vi "darksider.vi"(8 "sum threshold":dbl, 9 "background":u16=1000, 10 "Frame Index start":i32=-1, 11 "Path":path) -> (0 "Edge 2":i32, 1 "Edge 1":i32, 2 "lateral position indexs":dbl[](array[numeric]), 3 "centroid":sgl[][](array[numeric]), 4 "Total Frames":i32, 6 "index of element":i32)   [LabVIEW 2021]
uses:
  <vilib>/Analysis/baseanly.llb/Mean (DBL).vi
  <vilib>/vision/NI_Vision_Development_Module.lvlib
  <vilib>/Analysis/NI_AALBase.lvlib
panel:
  out "lateral position indexsy":dbl[](array[numeric])
  out "size(s)":i32
  out "Waveform Graph 2":sgl[](graph)
  out "Particle Reports (Pixels)":T1(array[cluster]) {"Orientation" format="%.2f"; "Dimensions"."Height" format="%.2f"; "Dimensions"."Width" format="%.2f"; "Center of Mass"."Y" format="%.2f"; "Center of Mass"."X" format="%.2f"; "Bounding Rect"."Bottom" format="%.2f"; "Bounding Rect"."Right" format="%.2f"; "Bounding Rect"."Top" format="%.2f"; "Bounding Rect"."Left" format="%.2f"; "Number of Holes" format="%.2f"; "Area" format="%.2f"}
  in  "Selection Values 2":T3(array[cluster])=[{"Measurement Parameter"=1, "Range Lower Value"=200.0, "Range Upper Value"=1848.0, "Range"=FALSE, "Measurement Type"=FALSE}] {"Measurement Parameter" items=["Center of Mass X", "Center of Mass Y", "First Pixel X", "First Pixel Y", "Bounding Rect Left", "Bounding Rect Top", "Bounding Rect Right", "Bounding Rect Bottom", "Max Feret Diameter Start X", "Max Feret Diameter Start Y", "Max Feret Diameter End X", "Max Feret Diameter End Y", "Max Horiz. Segment Length Left", "Max Horiz. Segment Length Right", "Max Horiz. Segment Length Row", "-", "Bounding Rect Width", "Bounding Rect Height", "Bounding Rect Diagonal", "Perimeter", "Convex Hull Perimeter", "Holes' Perimeter", "Max Feret Diameter", "Equivalent Ellipse Major Axis", "Equivalent Ellipse Minor Axis", "Equivalent Ellipse Minor Axis (Feret)", "Equivalent Rect Long Side", "Equivalent Rect Short Side", "Equivalent Rect Diagonal", "Equivalent Rect Short Side (Feret)", "Average Horiz. Segment Length", "Average Vert. Segment Length", "Hydraulic Radius", "Waddel Disk Diameter", "-", "Area", "Holes' Area", "Particle & Holes' Area", "Convex Hull Area", "Image Area", "-", "Number of Holes", "Number of Horiz. Segments", "Number of Vert. Segments", "-", "Orientation", "Max Feret Diameter Orientation", "-", "% Area/Image Area", "% Area/(Particle & Holes' Area)", "Ratio of Equivalent Ellipse Axes", "Ratio of Equivalent Rect Sides", "-", "Elongation Factor", "Compactness Factor", "Heywood Circularity Factor", "Type Factor", "-", "Sum X", "Sum Y", "Sum XX", "Sum XY", "Sum YY", "Sum XXX", "Sum XXY", "Sum XYY", "Sum YYY", "-", "Moment of Inertia XX", "Moment of Inertia XY", "Moment of Inertia YY", "Moment of Inertia XXX", "Moment of Inertia XXY", "Moment of Inertia XYY", "Moment of Inertia YYY", "Norm. Moment of Inertia XX", "Norm. Moment of Inertia XY", "Norm. Moment of Inertia YY", "Norm. Moment of Inertia XXX", "Norm. Moment of Inertia XXY", "Norm. Moment of Inertia XYY", "Norm. Moment of Inertia YYY", "Hu Moment 1", "Hu Moment 2", "Hu Moment 3", "Hu Moment 4", "Hu Moment 5", "Hu Moment 6", "Hu Moment 7"]; "Range Lower Value" format="%.2f"; "Range Upper Value" format="%.2f"}
  out "Waveform Chart":i32[](graph)
  out "yi":dbl[](array[numeric]) format="%_6g"
  out "time":dbl
  out "Waveform Graph":dbl[][](graph)
  out "Numeric":i32
  out "Frame Index":i32=-1
  in  "Connectivity 4/8":bool=TRUE
  out "sum 2":u16
  out "sum":i32
  out "Y Centroid":sgl
  out "X Centroid":sgl
  in  "Selection Values":T3(array[cluster])=[{"Measurement Parameter"=48, "Range Lower Value"=10.0, "Range Upper Value"=100.0, "Range"=FALSE, "Measurement Type"=FALSE}] {"Measurement Parameter" items=["Center of Mass X", "Center of Mass Y", "First Pixel X", "First Pixel Y", "Bounding Rect Left", "Bounding Rect Top", "Bounding Rect Right", "Bounding Rect Bottom", "Max Feret Diameter Start X", "Max Feret Diameter Start Y", "Max Feret Diameter End X", "Max Feret Diameter End Y", "Max Horiz. Segment Length Left", "Max Horiz. Segment Length Right", "Max Horiz. Segment Length Row", "-", "Bounding Rect Width", "Bounding Rect Height", "Bounding Rect Diagonal", "Perimeter", "Convex Hull Perimeter", "Holes' Perimeter", "Max Feret Diameter", "Equivalent Ellipse Major Axis", "Equivalent Ellipse Minor Axis", "Equivalent Ellipse Minor Axis (Feret)", "Equivalent Rect Long Side", "Equivalent Rect Short Side", "Equivalent Rect Diagonal", "Equivalent Rect Short Side (Feret)", "Average Horiz. Segment Length", "Average Vert. Segment Length", "Hydraulic Radius", "Waddel Disk Diameter", "-", "Area", "Holes' Area", "Particle & Holes' Area", "Convex Hull Area", "Image Area", "-", "Number of Holes", "Number of Horiz. Segments", "Number of Vert. Segments", "-", "Orientation", "Max Feret Diameter Orientation", "-", "% Area/Image Area", "% Area/(Particle & Holes' Area)", "Ratio of Equivalent Ellipse Axes", "Ratio of Equivalent Rect Sides", "-", "Elongation Factor", "Compactness Factor", "Heywood Circularity Factor", "Type Factor", "-", "Sum X", "Sum Y", "Sum XX", "Sum XY", "Sum YY", "Sum XXX", "Sum XXY", "Sum XYY", "Sum YYY", "-", "Moment of Inertia XX", "Moment of Inertia XY", "Moment of Inertia YY", "Moment of Inertia XXX", "Moment of Inertia XXY", "Moment of Inertia XYY", "Moment of Inertia YYY", "Norm. Moment of Inertia XX", "Norm. Moment of Inertia XY", "Norm. Moment of Inertia YY", "Norm. Moment of Inertia XXX", "Norm. Moment of Inertia XXY", "Norm. Moment of Inertia XYY", "Norm. Moment of Inertia YYY", "Hu Moment 1", "Hu Moment 2", "Hu Moment 3", "Hu Moment 4", "Hu Moment 5", "Hu Moment 6", "Hu Moment 7"]; "Range Lower Value" format="%.2f"; "Range Upper Value" format="%.2f"}
  in  "Fill Holes? (F)":bool
  in  "Reject Border? (F)":bool
  in  "Keep/Remove Particles (F)":bool
  out "Centroid 3":cluster{"X Centroid":sgl, "Y Centroid":sgl} {"Y Centroid" format="%.2f"; "X Centroid" format="%.2f"}
  out "Number of Particles":i32
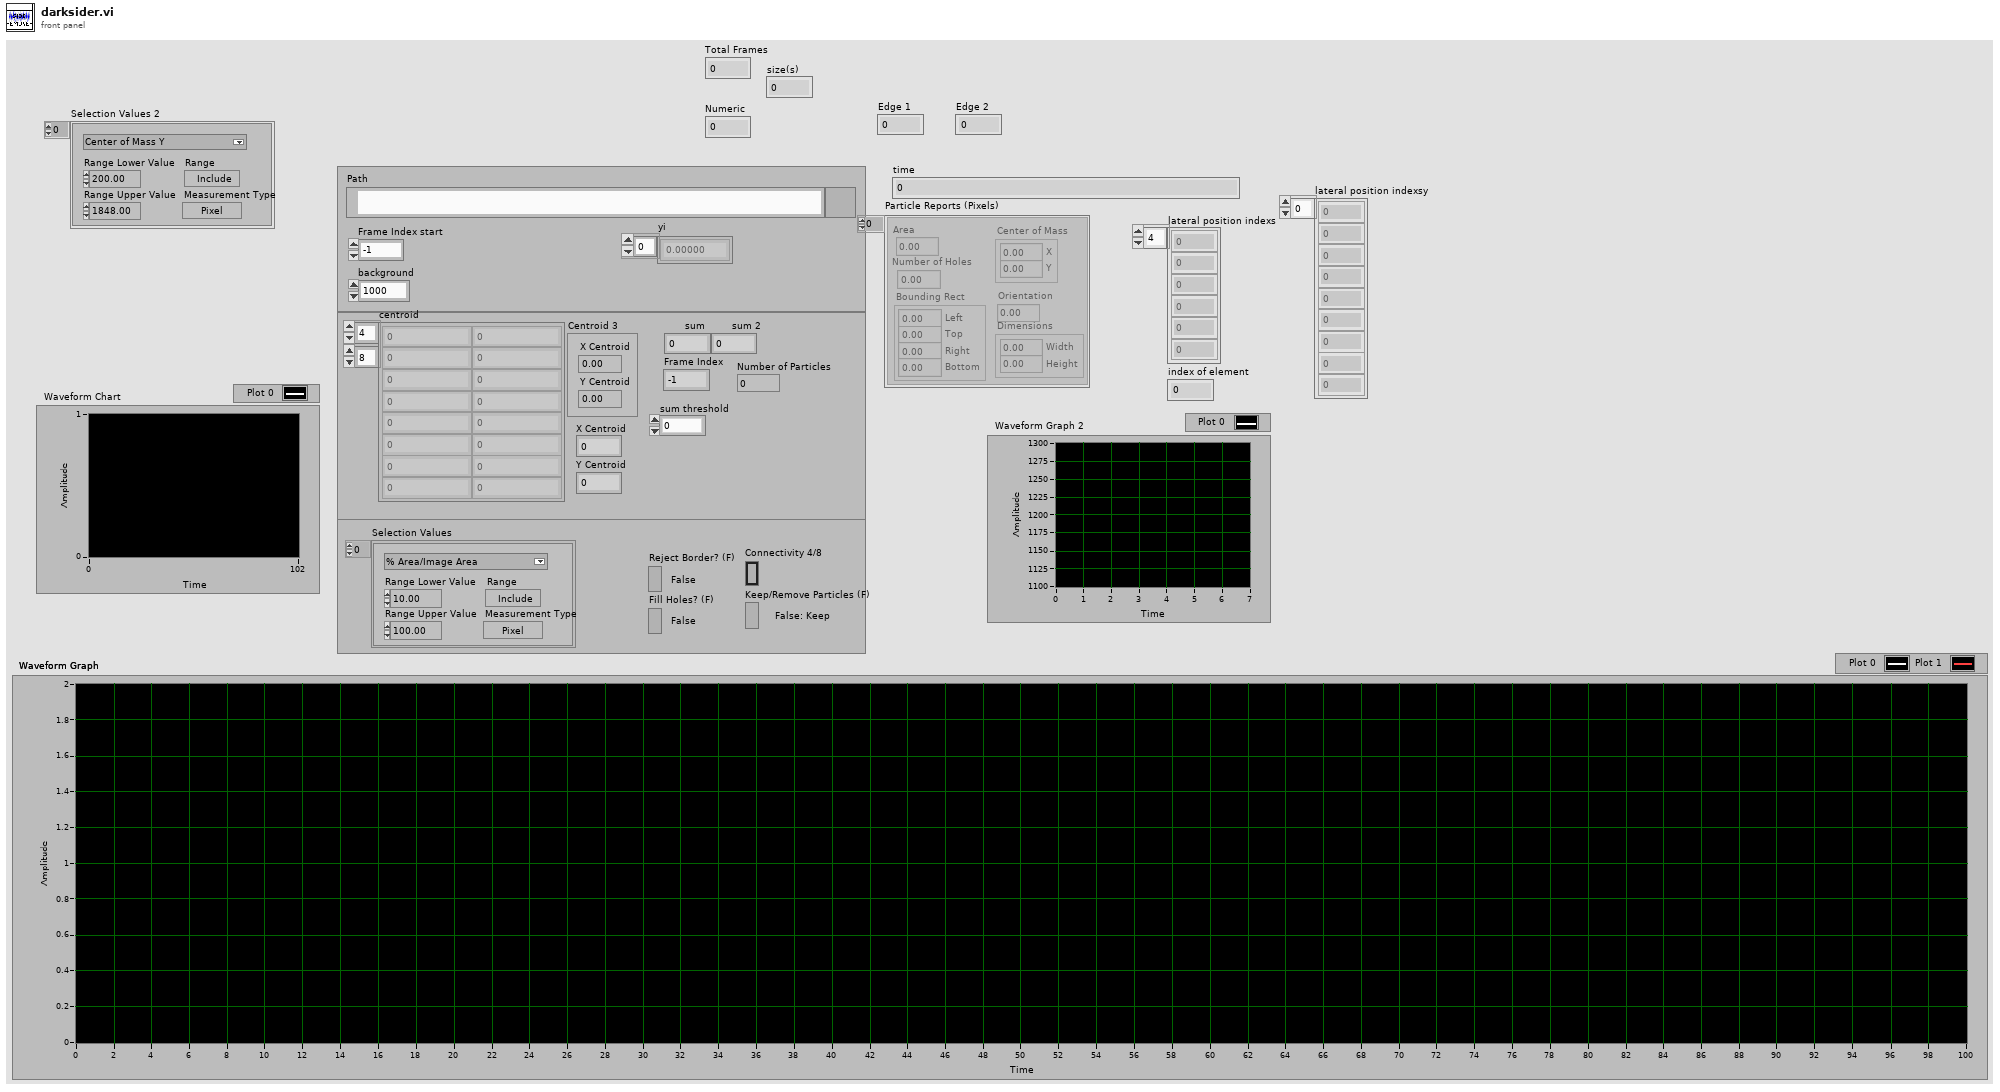
[diagram p1: front panel]
types:
  T1 = cluster{"Area":dbl, "Number of Holes":dbl, "Bounding Rect":cluster{"Left":dbl, "Top":dbl, "Right":dbl, "Bottom":dbl}, "Center of Mass":cluster{"X":dbl, "Y":dbl}, "Orientation":dbl, "Dimensions":cluster{"Width":dbl, "Height":dbl}}[]
  T2 = typedef "Particle Parameters" = i32
  T3 = cluster{"Measurement Parameter":T2, "Range Lower Value":dbl, "Range Upper Value":dbl, "Range":bool, "Measurement Type":bool}[]
  T4 = typedef "Image Type" = u32
  T5 = typedef "IMAQ Image.ctl" = refnum<image>
  T6 = cluster{"Particle Reports (Pixels)[0]":cluster{"Area":dbl, "Number of Holes":dbl, "Bounding Rect":cluster{"Left":dbl, "Top":dbl, "Right":dbl, "Bottom":dbl}, "Center of Mass":cluster{"X":dbl, "Y":dbl}, "Orientation":dbl, "Dimensions":cluster{"Width":dbl, "Height":dbl}}, "Particle Reports (Pixels)[1]":cluster{"Area":dbl, "Number of Holes":dbl, "Bounding Rect":cluster{"Left":dbl, "Top":dbl, "Right":dbl, "Bottom":dbl}, "Center of Mass":cluster{"X":dbl, "Y":dbl}, "Orientation":dbl, "Dimensions":cluster{"Width":dbl, "Height":dbl}}, "Particle Reports (Pixels)[2]":cluster{"Area":dbl, "Number of Holes":dbl, "Bounding Rect":cluster{"Left":dbl, "Top":dbl, "Right":dbl, "Bottom":dbl}, "Center of Mass":cluster{"X":dbl, "Y":dbl}, "Orientation":dbl, "Dimensions":cluster{"Width":dbl, "Height":dbl}}, "Particle Reports (Pixels)[3]":cluster{"Area":dbl, "Number of Holes":dbl, "Bounding Rect":cluster{"Left":dbl, "Top":dbl, "Right":dbl, "Bottom":dbl}, "Center of Mass":cluster{"X":dbl, "Y":dbl}, "Orientation":dbl, "Dimensions":cluster{"Width":dbl, "Height":dbl}}, "Particle Reports (Pixels)[4]":cluster{"Area":dbl, "Number of Holes":dbl, "Bounding Rect":cluster{"Left":dbl, "Top":dbl, "Right":dbl, "Bottom":dbl}, "Center of Mass":cluster{"X":dbl, "Y":dbl}, "Orientation":dbl, "Dimensions":cluster{"Width":dbl, "Height":dbl}}, "Particle Reports (Pixels)[5]":cluster{"Area":dbl, "Number of Holes":dbl, "Bounding Rect":cluster{"Left":dbl, "Top":dbl, "Right":dbl, "Bottom":dbl}, "Center of Mass":cluster{"X":dbl, "Y":dbl}, "Orientation":dbl, "Dimensions":cluster{"Width":dbl, "Height":dbl}}, "Particle Reports (Pixels)[6]":cluster{"Area":dbl, "Number of Holes":dbl, "Bounding Rect":cluster{"Left":dbl, "Top":dbl, "Right":dbl, "Bottom":dbl}, "Center of Mass":cluster{"X":dbl, "Y":dbl}, "Orientation":dbl, "Dimensions":cluster{"Width":dbl, "Height":dbl}}, "Particle Reports (Pixels)[7]":cluster{"Area":dbl, "Number of Holes":dbl, "Bounding Rect":cluster{"Left":dbl, "Top":dbl, "Right":dbl, "Bottom":dbl}, "Center of Mass":cluster{"X":dbl, "Y":dbl}, "Orientation":dbl, "Dimensions":cluster{"Width":dbl, "Height":dbl}}, "Particle Reports (Pixels)[8]":cluster{"Area":dbl, "Number of Holes":dbl, "Bounding Rect":cluster{"Left":dbl, "Top":dbl, "Right":dbl, "Bottom":dbl}, "Center of Mass":cluster{"X":dbl, "Y":dbl}, "Orientation":dbl, "Dimensions":cluster{"Width":dbl, "Height":dbl}}}
  T7 = cluster{"Area":dbl, "Number of Holes":dbl, "Bounding Rect":cluster{"Left":dbl, "Top":dbl, "Right":dbl, "Bottom":dbl}, "Center of Mass":cluster{"X":dbl, "Y":dbl}, "Orientation":dbl, "Dimensions":cluster{"Width":dbl, "Height":dbl}}
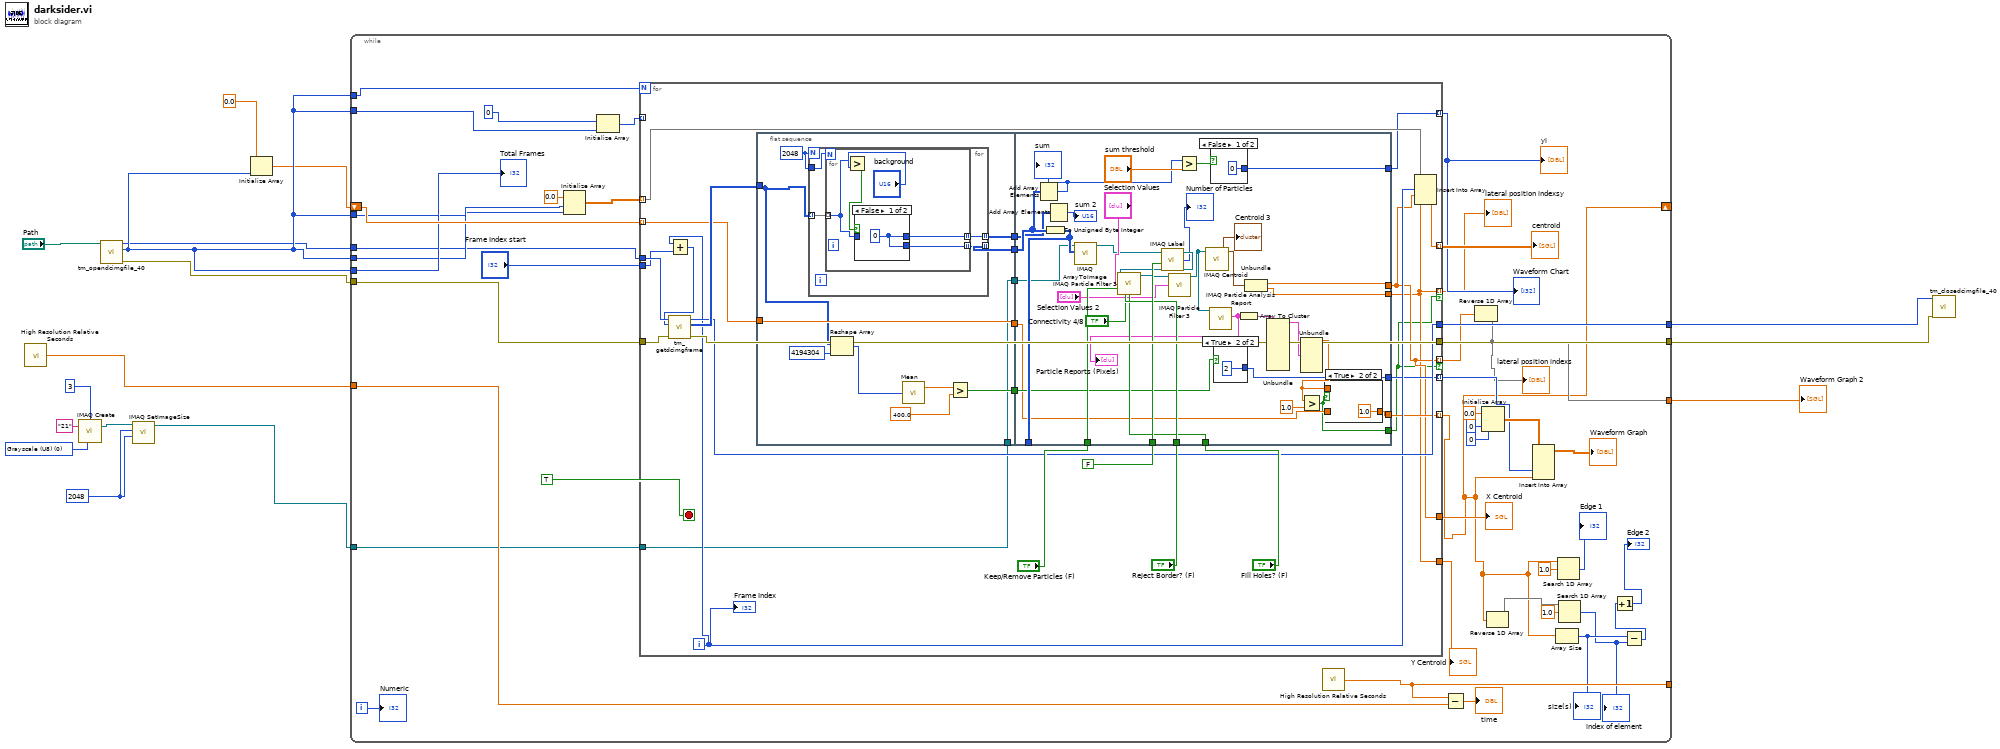
[diagram p0: block diagram]
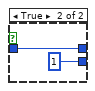
[diagram p2: hidden frame]
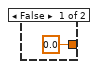
[diagram p3: hidden frame]
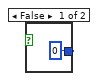
[diagram p4: hidden frame]
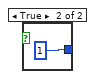
[diagram p5: hidden frame]
diagram:
  w14 = T4 0 items=["Grayscale (U8)", "Grayscale (I16)", "Grayscale (SGL)", "Complex (CSG)", "RGB (U32)", "HSL (U32)", "RGB (U64)", "Grayscale (U16)"] ("Image Type")
  w13 = 2048 ("X Resolution")
  n1 = call <vilib>:"High Resolution Relative Seconds.vi"() -> ("relative seconds"=w9:dbl)
  n2 = call "IMAQ Create"("Border Size"=3, "Image Name"="21", "Image Type"=w14) -> ("New Image"=w12:T5)  [unwired: 2 in, 1 out]
  n3 = call <userlib>:"tm_opendcimgfile_40.vi"("Path"="Path") -> ("error out"=w7:errorcluster, "Total Frames"=w11:i32, "File Handle"=w6:u32)  [unwired: 8 in]
  n4 = call "IMAQ SetImageSize"("Y Resolution"=w13, "X Resolution"=w13, "Image"=w12) -> ("Image Out"=w8:T5)  [unwired: 2 in, 1 out]
  n5 = Initialize Array(0.0 ("element"), w11) -> (w2:dbl[])
  n6 = while {
    tunnel: [w57] -> w4
    tunnel: [w58] -> w5
    tunnel: w9 -> [w46]
    tunnel: [w47] -> _
    shift-right: [w20] -> _
    shift-left: w2 -> [w38]
    tunnel: [w21] -> w3
    tunnel: w8 -> [w37]
    tunnel: w7 -> [w36]
    tunnel: w11 -> [w35]
    tunnel: w11 -> [w34]
    tunnel: w11 -> [w33]
    tunnel: w11 -> [w32]
    tunnel: w11 -> [w31]
    tunnel: w6 -> [w30]
    i -> [w48]
    stop <- TRUE ("stop") stop-if-true
    n7 = Initialize Array(0.0 ("element"), w32, w31) -> (w52:dbl[][])
    n8 = Initialize Array(0 ("dimension size"), w33) -> (w50:i32[])
    n9 = for {
      N: w35 -> [_]
      tunnel: w36 -> [w79]
      tunnel: "Frame Index start" -> [w71]
      tunnel: w30 -> [w78]
      tunnel: [w77] -> w58
      tunnel: [w73] -> w57
      tunnel: [w62] -> w56
      tunnel: [w61] -> w55
      tunnel: [w74] -> w54 mode=indexing
      tunnel: w52 -> [w75] mode=indexing
      tunnel: w50 -> [_] mode=indexing
      tunnel: [w69] -> w29 mode=indexing
      tunnel: [w67] -> w40 mode=indexing
      tunnel: w38 -> [w65] mode=indexing
      tunnel: [w64] -> w20 mode=indexing
      tunnel: [w62] -> w22 mode=indexing if=w60
      tunnel: w37 -> [w63]
      tunnel: [w61] -> w17 mode=indexing if=w60
      i -> [w72]
      n10 = Add(x=w72, y=w71) -> (x+y=w70:i32)
      n11 = call <userlib>:"tm_getdcimgframe.vi"("error in (no error)"=w79, "Frame Index"=w70, "File Handle in"=w78) -> ("error out"=w77:errorcluster, "Data"=w76:u16[][], "File Handle out"=w73:u32)  [unwired: 5 in, 1 out]
      n12 = flat-sequence {
        tunnel: [w97] -> w86
        tunnel: [w96] -> w85
        tunnel: [w88] -> w84
        tunnel: w76 -> [w87]
        tunnel: [w90] -> w68
        tunnel: [w89] -> w66
        tunnel: w65 -> [w89]
        tunnel: w63 -> [w88]
        tunnel: w86 -> [w131]
        tunnel: w85 -> [w132]
        tunnel: w84 -> [w128]
        tunnel: FALSE ("Connectivity 4/8 (8)") -> [w143]
        tunnel: "Keep/Remove Particles (F)" -> [w139]
        tunnel: "Reject Border? (F)" -> [w138]
        tunnel: "Fill Holes? (F)" -> [w137]
        tunnel: [w135] -> w62
        tunnel: [w134] -> w61
        tunnel: [w133] -> _
        tunnel: [w124] -> w69
        tunnel: w68 -> [w120]
        tunnel: [w119] -> w67
        tunnel: w66 -> [w113]
        tunnel: [w112] -> w64
        tunnel: [w110] -> w60
        frame #0 {
          w95 = 2048
          n13 = for {
            N: w95 -> [_]
            tunnel: w87 -> [w101] mode=indexing
            tunnel: [w100] -> w97 mode=indexing
            tunnel: [w99] -> w96 mode=indexing
            tunnel: w95 -> [w98]
            n14 = for {
              N: w98 -> [_]
              tunnel: w101 -> [w104] mode=indexing
              tunnel: [w103] -> w100 mode=indexing
              tunnel: [w102] -> w99 mode=indexing
              n15 = Greater?(x=w104, y="background") -> (0:w105:bool)
              n16 = case shown="False" w105 {
                tunnel: w104 -> [_ w109]
                tunnel: [w107 w109] -> w103
                tunnel: [w107 1] -> w102
                frame False {
                  w107 = u16 0 ("Numeric")
                }
                frame True {
                }
              }
            }
          }
          n17 = Reshape Array(w87, 4194304 ("dimension size")) -> (w93:u16[])
          n18 = call-poly <vilib>:"Mean.vi"("X"=w93) -> ("mean"=w94:dbl)  [unwired: 1 out]
          n19 = Greater?(x=w94, y=400.0) -> (0:w90:bool)
        }
        frame #1 {
          n20 = Add Array Elements(numeric array=w132) -> (sum=w126:i32)
          "sum" <- w126
          n21 = To Unsigned Byte Integer(number=w132) -> (unsigned 8bit integer=w133:u8[][])
          n22 = Add Array Elements(numeric array=w131) -> (sum=→"sum 2":u16)
          n23 = call "IMAQ ArrayToImage"("Image Pixels (U8)"=w133, "Image"=w128) -> ("Image Out"=w123:T5)  [unwired: 8 in, 1 out]
          n24 = call "IMAQ Label"("Connectivity 4/8 (8)"=w143, "Image Src"=w123) -> ("Number of Particles"=→"Number of Particles":i32, "Image Dst Out"=w142:T5)  [unwired: 2 in, 1 out]
          n25 = call "IMAQ Particle Filter 3"("Image Src"=w142, "Connectivity 4/8 (8)"="Connectivity 4/8", "Selection Values"="Selection Values", "Keep/Remove Particles (F)"=w139, "Reject Border? (F)"=w138, "Fill Holes? (F)"=w137) -> ("Image Dst Out"=w122:T5)  [unwired: 7 in, 2 out]
          n26 = call "IMAQ Particle Filter 3"("Image Src"=w122, "Selection Values"="Selection Values 2") -> ("Image Dst Out"=w118:T5)  [unwired: 11 in, 2 out]
          n27 = Greater?(x=w126, y="sum threshold") -> (0:w125:bool)
          n28 = call "IMAQ Centroid"("Image"=w118) -> ("Centroid"=w141:cluster{"X Centroid":sgl, "Y Centroid":sgl})  [unwired: 3 in, 1 out]
          "Centroid 3" <- w141
          n29 = call "IMAQ Particle Analysis Report"("Image"=w118) -> ("Particle Reports (Pixels)"=w117:T1)  [unwired: 5 in, 5 out]
          "Particle Reports (Pixels)" <- w117
          n30 = case shown="False" w125 {
            tunnel: [0 1] -> w124
            frame False {
            }
            frame True {
            }
          }
          n31 = case shown="True" w120 {
            tunnel: [0 2] -> w119
            frame False {
            }
            frame True {
            }
          }
          n32 = Array To Cluster(array=w117) -> (cluster=w116:T6)
          n33 = Unbundle(w141) -> ("X Centroid"=w135:sgl, "Y Centroid"=w134:sgl)
          n34 = Unbundle(w116) -> ("Particle Reports (Pixels)[0]"=w115:T7)  [unwired: 8 out]
          n35 = Unbundle(w115) -> ("Area"=w111:dbl)  [unwired: 5 out]
          n36 = Greater?(x=w111, y=1.0) -> (0:w110:bool)
          n37 = case shown="True" w110 {
            tunnel: w113 -> [_ _]
            tunnel: [0.0 ("Area") 1.0 ("Area")] -> w112
            tunnel: w111 -> [_ _]
            frame False {
            }
            frame True {
            }
          }
        }
      }
      n38 = Insert Into Array(array=w75, index=w72, new element #1=w62, new element #2=w61) -> (w74:dbl[])
      "Frame Index" <- w72
    }
    "X Centroid" <- w56
    "Y Centroid" <- w55
    "centroid" <- w54
    "yi" <- w29
    "Waveform Chart" <- w29
    "lateral position indexsy" <- w17
    n39 = call <vilib>:"High Resolution Relative Seconds.vi"() -> ("relative seconds"=w47:dbl)
    n40 = Subtract(x=w47, y=w46) -> (x-y=→"time":dbl)
    n41 = Reverse 1D Array(array=w22) -> (reversed array=w21:sgl[])
    "lateral position indexs" <- w21
    n42 = Initialize Array(0.0 ("element"), 0 ("dimension size"), 0 ("dimension size")) -> (w41:dbl[][])
    n43 = Reverse 1D Array(array=w20) -> (reversed array=w28:dbl[])
    n44 = Insert Into Array(array=w41, new element #1=w40, new element #2=w20) -> (→"Waveform Graph":dbl[][])  [unwired: 2 in]
    n45 = Array Size(array=w20) -> (size(s)=w24:i32)
    "size(s)" <- w24
    n46 = Search 1D Array(1D array=w20, element=1.0) -> (index of element=→"Edge 1":i32)  [unwired: 1 in]
    n47 = Search 1D Array(1D array=w28, element=1.0) -> (index of element=w23:i32)  [unwired: 1 in]
    "index of element" <- w23
    n48 = Subtract(x=w24, y=w23) -> (x-y=w19:i32)
    n49 = Increment(x=w19) -> (x+1=→"Edge 2":i32)
    "Numeric" <- w48
    "Total Frames" <- w34
  }
  "Waveform Graph 2" <- w3
  n50 = call <userlib>:"tm_closedcimgfile_40.vi"("error in (no error)"=w5, "File Handle"=w4) -> ()  [unwired: 9 in, 1 out]
